vi "Query with 2D String Result.vi"(8 "error in (no error)":errorcluster, 10 "Query string":string, 11 "mysql in":refnum<class "mysql.lvclass">) -> (0 "error out":errorcluster, 2 "Result":string[][](array[string]), 3 "mysql out":refnum<class "mysql.lvclass">)   [LabVIEW 2020, in "mysql.lvlib" / "mysql.lvclass"]
uses:
  mysql.lvclass
  d09922f1-abe6-4b23-a0e6-d86b877a536f.vi
  private/Mysql command.vi
  private/Mysql data reader 2D string.vi
  private/ping connection and reopen if needed.vi
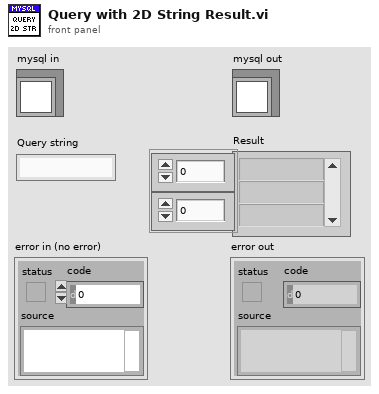
[diagram p1: front panel]
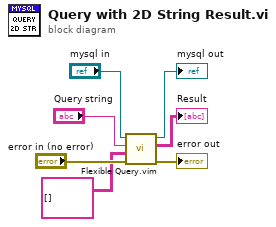
[diagram p0: block diagram]
diagram:
  n1 = call "Flexible Query.vim"("error in (no error)"="error in (no error)", "Type in"=string[][] [] ("Result 2"), "Query string"="Query string", "mysql in"="mysql in") -> ("error out"=→"error out":errorcluster, "Result"=→"Result":string[][], "mysql out"=→"mysql out":refnum<class "mysql.lvclass">)  [unwired: 5 in]
